vi "Test_allsw_IPK_Linux_Moblise.vi"() -> (0 "pass":bool)   [LabVIEW 2020]
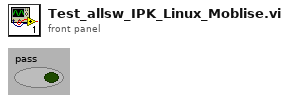
[diagram p1: front panel]
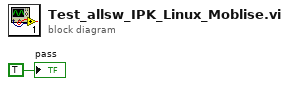
[diagram p0: block diagram]
diagram:
  "pass" <- TRUE
